vi "Set Control Value Signaling.vi"(6 "value":variant, 8 "error in (no error)":errorcluster, 9 "label":string, 10 "object class":T1, 11 "Panel":refnum<vi>) -> (0 "error out":errorcluster, 3 "Panel out":refnum<vi>)   [LabVIEW 2018, in "NISAST VI Scripting.lvlib" / "VI.lvlib" / "Front Panel.lvlib"]
uses:
  Front Panel.lvlib
  Type Define/Object Class.ctl
  Agilent N5232A PNA-L/Labview Driver/Keysight PNA Series/express/Utility/StudioHelper/Common/VI Scripting/Type Define/Type Define.lvlib
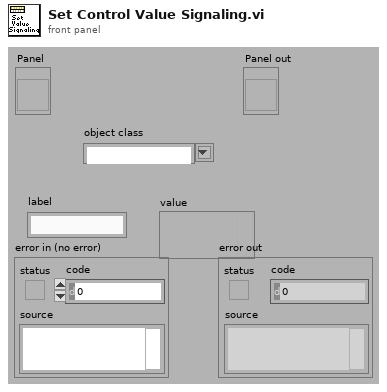
[diagram p1: front panel]
types:
  T1 = typedef "NISAST VI Scripting.lvlib/Type Define.lvlib/Object Class.ctl" = string
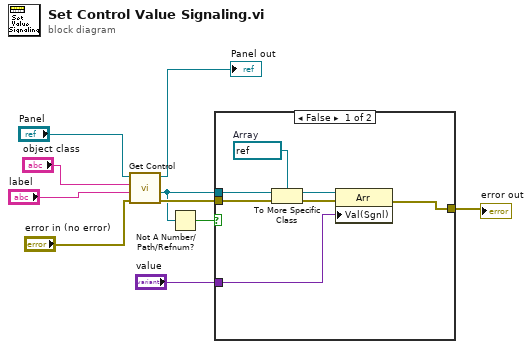
[diagram p0: block diagram]
diagram:
  n1 = call "Get Control.vi"("error in (no error)"="error in (no error)", "label"="label", "object class"="object class", "Panel"="Panel") -> ("error out"=w10:errorcluster, "first control"=w8:refnum<vi>, "Panel out"=→"Panel out":refnum<vi>)  [unwired: 5 out]
  n2 = Not A Number/Path/Refnum?(number/path/refnum=w8) -> (NaN/Path/Refnum?=w9:bool)
  n3 = case shown="False" w9 {
    tunnel: w8 -> [w17 _]
    tunnel: w10 -> [w16 w18]
    tunnel: [w12 w18] -> w5
    tunnel: "value" -> [w11 _]
    frame False {
      w15 = refnum<vi> refnum  # Array
      n4 = To More Specific Class(target class=w15, reference=w17, error in=w16) -> (specific class reference=w14:refnum<vi>, error out=w13:errorcluster)
      n5 = property class="Arr"(reference=w14, error in=w13, "Val(Sgnl)"=w11) -> (error out=w12:errorcluster)  [unwired: 1 out]
    }
    frame True {
    }
  }
  "error out" <- w5
